vi "Change.vi"(6 "OldVal":variant, 8 "error in (no error)":errorcluster, 9 "NewVal":variant, 10 "Control Index":i32=-1, 11 "All Queue in":T1) -> (0 "error out":errorcluster, 1 "Redo Enable":bool, 2 "Undo Enable":bool, 3 "All Queue out":T1)   [LabVIEW 2015, in "UndoLibrary.lvlib"]
doc: "This VI stores the changes produced in the controls. The maximum number of change is corresponding to the size of the buffer."
uses:
  UndoLibrary.lvlib
  Controls/cluster_All Queue.ctl
  Controls/cluster_Control Value.ctl
  <vilib>/Utility/error.llb/Error Cluster From Error Code.vi
  <vilib>/ErrorRing/Error Ring.xnode
  QueueOperations/QueueOperations.lvlib
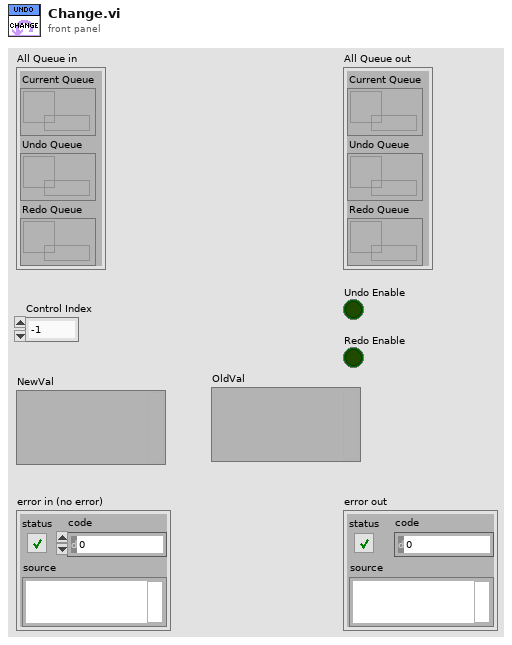
[diagram p1: front panel]
types:
  T1 = typedef "UndoLibrary.lvlib/cluster_All Queue.ctl" = cluster{"Current Queue":refnum<queue>, "Undo Queue":refnum<queue>, "Redo Queue":refnum<queue>}
  T2 = typedef "UndoLibrary.lvlib/cluster_Control Value.ctl" = cluster{"Index":i32, "Variant Data":variant}
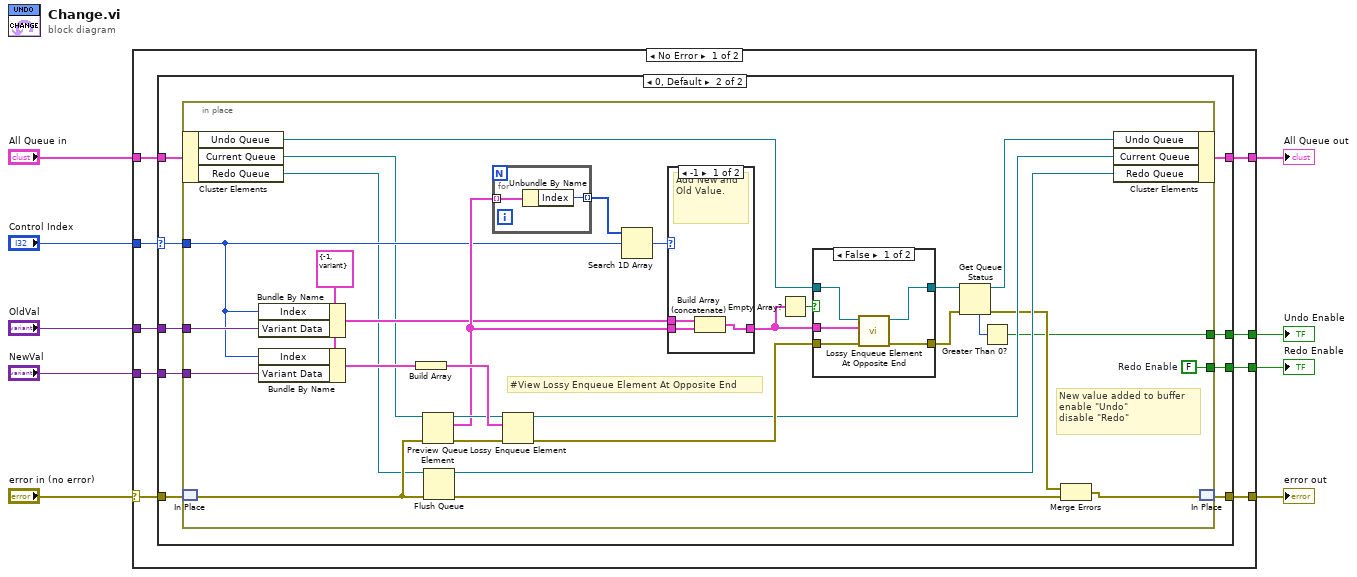
[diagram p0: block diagram]
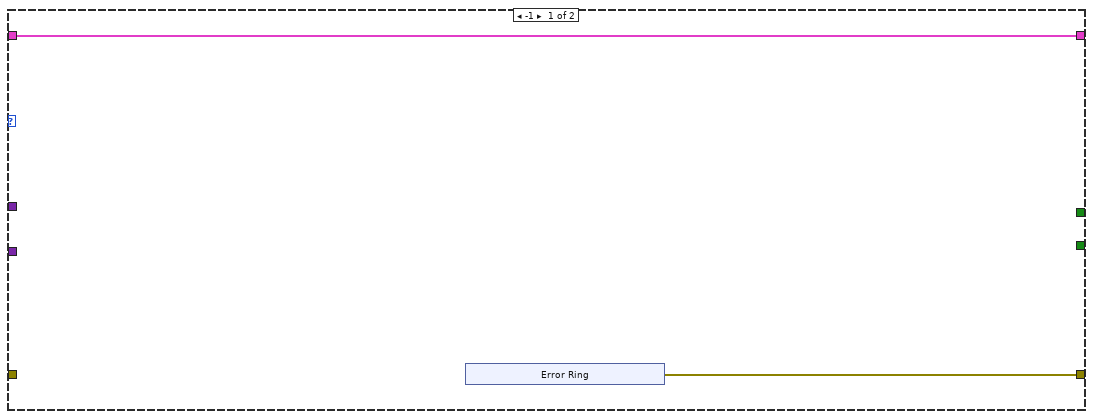
[diagram p2: hidden frame]
diagram:
  n1 = case shown="No Error" "error in (no error)" {
    selector: "error in (no error)" -> [w15 w78]
    tunnel: "OldVal" -> [w18 _]
    tunnel: "NewVal" -> [w17 _]
    tunnel: "Control Index" -> [w16 _]
    tunnel: "All Queue in" -> [w13 w77]
    tunnel: [w12 w77] -> w5
    tunnel: [w14 w78] -> w3
    tunnel: [w11 _] -> w2
    tunnel: [w10 _] -> w1
    frame No Error {
      n2 = case shown="0, Default" w16 {
        selector: w16 -> [_ w31]
        tunnel: w18 -> [_ w33]
        tunnel: w17 -> [_ w32]
        tunnel: w15 -> [_ w30]
        tunnel: [w19 w29] -> w14
        tunnel: w13 -> [w20 w28]
        tunnel: [w20 w27] -> w12
        tunnel: [_ w26] -> w11
        tunnel: [_ w25] -> w10
        frame -1 {
          n3 = xnode "Error Ring"() -> ("error out"=w19:errorcluster)
        }
        frame 0, Default {
          n4 = in-place {
            in-place-border: w33 -> [w55]
            in-place-border: w32 -> [w54]
            in-place-border: w31 -> [w50]
            in-place-border: [w35] -> w26
            in-place-border: [w34] -> w25
            w34 = FALSE  # Redo Enable
            w59 = T2 {"Index"=-1, "Variant Data"=variant} ("Control Value")
            # "New value added to buffer\nenable \"Undo\"\ndisable \"Redo\""
            # "#View Lossy Enqueue Element At Opposite End"
            n5 = in-place-cluster #1(w28) -> ("Undo Queue"=w45:refnum<queue>, "Current Queue"=w44:refnum<queue>, "Redo Queue"=w43:refnum<queue>)
            n6 = in-place-match #2(w30) -> (w47:errorcluster)
            n7 = Bundle By Name(cluster=w59, "Index"=w50, "Variant Data"=w55) -> (w56:T2)
            n8 = Bundle By Name(cluster=w59, "Index"=w50, "Variant Data"=w54) -> (w51:T2)
            n9 = Build Array(w51) -> (w63:T2[])
            n10 = Preview Queue Element(queue=w44, error in (no error)=w47) -> (queue out=w61:refnum<queue>, element=w60:T2[], error out=w62:errorcluster)  [unwired: 1 in, 1 out]
            n11 = Flush Queue(queue=w43, error in (no error)=w47) -> (queue out=w38:refnum<queue>, error out=w49:errorcluster)  [unwired: 1 out]
            n12 = for {
              tunnel: [w65] -> w57 mode=indexing
              tunnel: w60 -> [w64] mode=indexing
              n13 = Unbundle By Name(w64) -> ("Index"=w65:i32)
            }
            n14 = Lossy Enqueue Element(queue=w61, element=w63, error in (no error)=w62) -> (queue out=w42:refnum<queue>, error out=w48:errorcluster)  [unwired: 2 out]
            n15 = Search 1D Array(1D array=w57, element=w50) -> (index of element=w58:i32)  [unwired: 1 in]
            n16 = case shown="-1" w58 {
              tunnel: w60 -> [w68 w69]
              tunnel: [w67 w69] -> w53
              tunnel: w56 -> [w66 _]
              frame -1 {
                # "Add New and Old Value."
                n17 = Build Array (concatenate)(w66, w68) -> (w67:T2[])
              }
              frame 0, Default {
                # "Add Only New Value."
              }
            }
            n18 = Empty Array?(array=w53) -> (empty?=w52:bool)
            n19 = case shown="False" w52 {
              tunnel: w45 -> [w74 w76]
              tunnel: [w71 w76] -> w41
              tunnel: w48 -> [w72 w75]
              tunnel: [w70 w75] -> w37
              tunnel: w53 -> [w73 _]
              frame False {
                n20 = call "Lossy Enqueue Element At Opposite End.vi"("error in (no error)"=w72, "element"=w73, "queue in"=w74) -> ("error out"=w70:errorcluster, "queue out"=w71:refnum<queue>)  [unwired: 5 in, 2 out]
              }
              frame True {
              }
            }
            n21 = Get Queue Status(queue=w41, error in (no error)=w37) -> (queue out=w40:refnum<queue>, error out=w36:errorcluster, # elements in queue=w39:i32)  [unwired: 1 in, 5 out]
            n22 = Greater Than 0?(x=w39) -> (x > 0?=w35:bool)
            n23 = Merge Errors(w36, w49) -> (w46:errorcluster)
            n24 = in-place-cluster #1("Undo Queue"=w40, "Current Queue"=w42, "Redo Queue"=w38) -> (w27:T1)
            n25 = in-place-match #2(w46) -> (w29:errorcluster)
          }
        }
      }
    }
    frame Error {
    }
  }
  "error out" <- w3
  "All Queue out" <- w5
  "Undo Enable" <- w2
  "Redo Enable" <- w1
